vi "Calculate time.vi"(8 "error in (no error)":errorcluster, 10 "Average time":dbl, 11 "Run Block in":refnum<class "Run Block.lvclass">) -> (0 "error out":errorcluster, 1 "Time":dbl, 2 "Number of scripts":u32, 3 "Run Block out":refnum<class "Run Block.lvclass">)   [LabVIEW 2020, in "Run Utilities.lvlib" / "Run Block.lvclass"]
doc: "Calculate number of scripts left in the shcedule and estimate time of the execution (in seconds) based on the average time"
uses:
  Run Block.lvclass
  Run Instance/Run Instance.lvclass
  Schedule/Schedule.lvclass
  Run Block.lvclass/Run Block.ctl
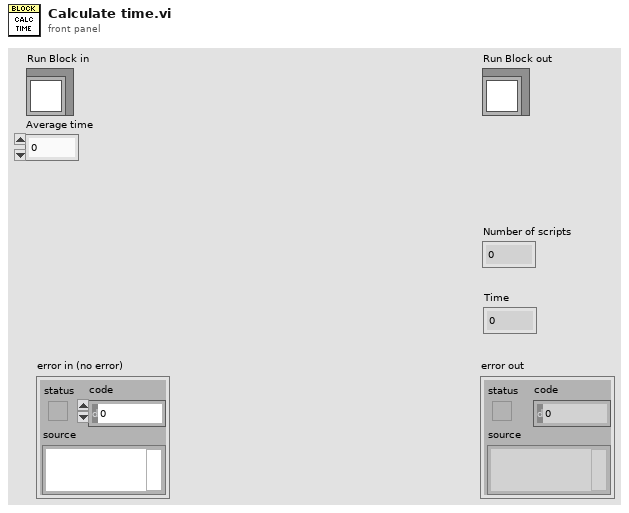
[diagram p1: front panel]
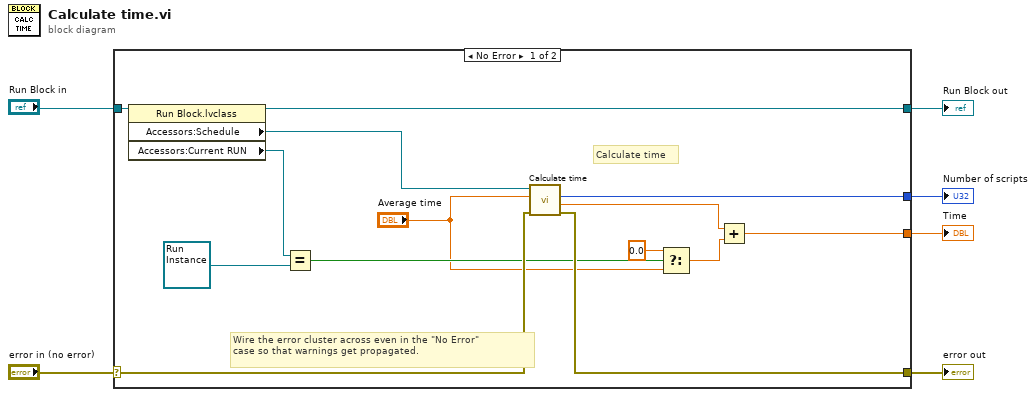
[diagram p0: block diagram]
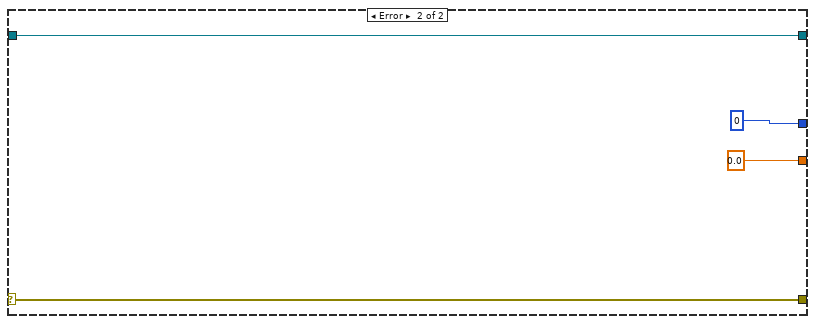
[diagram p2: hidden frame]
diagram:
  n1 = case shown="No Error" "error in (no error)" {
    selector: "error in (no error)" -> [w16 w24]
    tunnel: [w20 w24] -> w5
    tunnel: [w18 w23] -> w1
    tunnel: "Run Block in" -> [w19 w23]
    tunnel: [w7 0.0] -> w4
    tunnel: [w8 u32 0 ("y")] -> w3
    frame No Error {
      # "Calculate time"
      # "Wire the error cluster across even in the \"No Error\"\ncase so that warnings get propagated."
      n2 = property class="Run Block.lvclass"(reference=w19) -> (reference out=w18:refnum<class "Run Block.lvclass">, "Accessors:Schedule"=w17:refnum<class "Schedule.lvclass">, "Accessors:Current RUN"=w15:refnum<class "Run Instance.lvclass">)  [unwired: 1 in, 1 out]
      n3 = Equal?(x=w15, y=refnum<class "Run Instance.lvclass"> refnum) -> (x = y?=w13:bool)
      n4 = call-dynamic "Calculate time.vi"("error in (no error)"=w16, "Average time"="Average time", "Schedule in"=w17) -> ("error out"=w20:errorcluster, "Time"=w9:dbl, "Number of scripts"=w8:u32)  [unwired: 5 in, 1 out]
      n5 = Select(t=0.0, s=w13, f="Average time") -> (s? t:f=w10:dbl)
      n6 = Add(x=w9, y=w10) -> (x+y=w7:dbl)
    }
    frame Error {
    }
  }
  "error out" <- w5
  "Time" <- w4
  "Number of scripts" <- w3
  "Run Block out" <- w1
